vi "distance.vi"(10 "X2":dbl[](array[numeric]), 11 "X1":dbl[](array[numeric])) -> (3 "d":dbl)   [LabVIEW 2009, in "LV_SLAM.lvlib"]
uses:
  LV_SLAM.lvlib
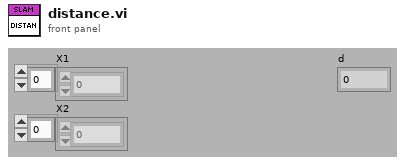
[diagram p1: front panel]
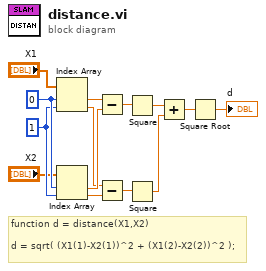
[diagram p0: block diagram]
diagram:
  w9 = 1 ("index")
  w10 = 0 ("index")
  # "function d = distance(X1,X2)\n\nd = sqrt( (X1(1)-X2(1))^2 + (X1(2)-X2(2))^2 );"
  n1 = Index Array(array="X1", index #1=w10, index #2=w9) -> (element #1=w6:dbl, element #2=w4:dbl)
  n2 = Index Array(array="X2", index #1=w10, index #2=w9) -> (element #1=w5:dbl, element #2=w3:dbl)
  n3 = Subtract(x=w6, y=w5) -> (x-y=w2:dbl)
  n4 = Subtract(x=w4, y=w3) -> (x-y=w1:dbl)
  n5 = Square(x=w2) -> (x^2=w14:dbl)
  n6 = Square(x=w1) -> (x^2=w13:dbl)
  n7 = Add(x=w14, y=w13) -> (x+y=w12:dbl)
  n8 = Square Root(x=w12) -> (sqrt(x)=→"d":dbl)
